vi "bilinear interpolation -- view.vi"() -> ()   [LabVIEW 2010]
uses:
  cursor winow.ctl
  <vilib>/event_ctls.llb/eventvkey.ctl
  cursor window action.ctl
  bylinear interpolation iiii- complex -- build matrix.vi
  Q -- check range -- i -- real.vi
  generate linear region.vi
  line -- complex.vi
  Q -- check range -- i -- integer.vi
  Q - not nan -- real.vi
  Q - not nan -- integer.vi
  Split file name.vi
  <vilib>/Utility/file.llb/Read From Spreadsheet File.vi
  <vilib>/Utility/file.llb/Read From Spreadsheet File (string).vi
  Q regex box.vi
  <vilib>/Analysis/Matrix/Numeric/Conversions/Array To Matrix.vi
  <vilib>/Analysis/Matrix/Numeric/Conversions/Array To Matrix - RA2.vi
  <vilib>/Analysis/baseanly.llb/Inverse Matrix.vi
  <vilib>/Analysis/baseanly.llb/Real Inverse Matrix.vi
  <vilib>/analysis/baseanly.llb/A x B.vi
  <vilib>/Analysis/baseanly.llb/Complex A x B.vi
panel:
  in  "number of segments":i32=3
  out "radius":dbl
  out "circle center":cdb
  in  "scale gauge: Plot: complex plane - filter":dbl(slide)=0.3 min=0.0 max=0.3 step=1e-05 scale=1e-05..0.3 scale format="%#_2g"
  out "Plot: complex plane - filter":cluster{dbl[], dbl[]}[](graph)=[{array[1630 elements], array[1630 elements]}, {[0.4066553079816637, 0.40327728987953354, 0.3931965089365436, 0.37657194509013175, 0.35366577764318885, 0.3248392505398343, 0.2905469753326207, 0.2513297616867779, 0.20780608848872892, 0.16066235006458904, 0.11064203133161113, 0.058533982596904274, 0.005159978916854432, -0.048638239786419776, -0.10201224346646971, -0.15412029220117648, -0.20414061093415437, -0.25128434935829436, -0.29480802255634325, -0.33402523620218605, -0.36831751140939956, -0.39714403851275415, -0.4200502059596971, -0.4366747698061089, -0.44675555074909884, -0.450133568851229, -0.44675555074909884, -0.4366747698061089, -0.420050205959697, -0.3971440385127541, -0.3683175114093995, -0.334025236202186, -0.29480802255634314, -0.25128434935829413, -0.20414061093415412, -0.15412029220117648, -0.10201224346646963, -0.04863823978641969, 0.005159978916854609, 0.05853398259690454, 0.11064203133161105, 0.160662350064589, 0.207806088488729, 0.25132976168677806, 0.2905469753326208, 0.3248392505398345, 0.35366577764318885, 0.3765719450901318, 0.3931965089365437, 0.40327728987953354], [-0.02173913043478265, 0.03195292977291478, 0.08479823411705473, 0.1359633805798755, 0.18464146423708142, 0.23006480263052065, 0.27151704257914155, 0.30834445749658657, 0.33996625704997624, 0.36588374657040623, 0.3856881917657815, 0.399067264704769, 0.40580996941485, 0.40580996941485, 0.39906726470476894, 0.3856881917657815, 0.36588374657040623, 0.33996625704997624, 0.30834445749658657, 0.2715170425791415, 0.23006480263052065, 0.18464146423708136, 0.1359633805798754, 0.08479823411705474, 0.03195292977291471, -0.02173913043478279, -0.07543119064248009, -0.12827649498662014, -0.17944164144944094, -0.22811972510664674, -0.273543063500086, -0.31499530344870685, -0.3518227183661519, -0.38344451791954165, -0.40936200743997164, -0.4291664526353468, -0.4425455255743343, -0.4492882302844153, -0.4492882302844153, -0.44254552557433424, -0.42916645263534686, -0.40936200743997153, -0.38344451791954154, -0.3518227183661518, -0.3149953034487067, -0.27354306350008567, -0.22811972510664671, -0.17944164144944075, -0.12827649498661992, -0.07543119064247988]}, {[-0.08588521013843603, -0.0794706021680707, -0.07305599419770535, -0.06664138622734002, -0.06022677825697468, -0.05381217028660934, -0.04739756231624401, -0.04098295434587867, -0.03456834637551333, -0.02815373840514799, -0.02173913043478265, -0.015324522464417317, -0.008909914494051985, -0.0024953065236866384, 0.003919301446678694, 0.01033390941704404, 0.016748517387409373, 0.023163125357774705, 0.029577733328140052, 0.035992341298505384], [0.4018255934561417, 0.35946912106704926, 0.31711264867795685, 0.2747561762888644, 0.23239970389977196, 0.19004323151067953, 0.14768675912158707, 0.10533028673249467, 0.06297381434340221, 0.020617341954309754, -0.02173913043478265, -0.06409560282387511, -0.10645207521296757, -0.14880854760206003, -0.19116501999115237, -0.23352149238024483, -0.2758779647693373, -0.31823443715842975, -0.3605909095475222, -0.40294738193661456]}, {[0.4018255934561417, 0.35946912106704926, 0.31711264867795685, 0.2747561762888644, 0.23239970389977196, 0.19004323151067953, 0.14768675912158707, 0.10533028673249467, 0.06297381434340221, 0.020617341954309754, -0.02173913043478265, -0.06409560282387511, -0.10645207521296757, -0.14880854760206003, -0.19116501999115237, -0.23352149238024483, -0.2758779647693373, -0.31823443715842975, -0.3605909095475222, -0.40294738193661456], [0.04240694926887073, 0.03599234129850539, 0.029577733328140055, 0.02316312535777472, 0.01674851738740938, 0.01033390941704404, 0.003919301446678708, -0.0024953065236866315, -0.008909914494051971, -0.01532452246441731, -0.02173913043478265, -0.028153738405147982, -0.034568346375513315, -0.04098295434587866, -0.047397562316243994, -0.05381217028660934, -0.06022677825697467, -0.06664138622734, -0.07305599419770535, -0.07947060216807068]}, {[-0.03480491194516355, -0.03153571549706419, -0.02826039650219348, -0.024981001928307045, -0.021699581290264596, -0.018418185369150124, -0.015138864930600241, -0.011863669443142526, -0.008594645797344487, -0.0053338370265733695, -0.002083281030167059, 0.0011549907001868857, 0.004378954350067313, 0.007586595047137542, 0.010775908120375176, 0.01394490035292599, 0.017091591227799845, 0.020214014165629166, 0.023310217753717, 0.02637826696560664], [-0.15235728022815603, -0.15264307469559787, -0.15284705845898403, -0.15296910403510236, -0.15300913514944053, -0.15296712678385516, -0.15284310519220728, -0.1526371478839546, -0.15234938357571062, -0.15197999211080082, -0.15152920434686656, -0.15099730201158656, -0.15038461752660615, -0.14969153379978473, -0.1489184839858907, -0.1480659512158939, -0.1471344682950244, -0.1461246173697867, -0.14503702956413708, -0.14387238458505142]}, {[-0.03913246135316176, -0.03478046636428151, -0.030420320964959106, -0.026054750104140326, -0.021686482121507648, -0.017318247042357023, -0.012952774871420701, -0.008592793886703221, -0.004241028934396603, 9.980027406010505e-05, 0.00442698086171163, 0.008737808481546538, 0.013029589006625965, 0.017299640213825143, 0.021545293460135825, 0.02576389535048096, 0.02995280939600055, 0.03410941766177122, 0.038231122402930216, 0.04231534768818167], [-0.19561963666378376, -0.19600008981485692, -0.19627163553875665, -0.19643410412824466, -0.19648739404574114, -0.19643147198678232, -0.19626637290083468, -0.19599219996945272, -0.19560912454179388, -0.1951173860275308, -0.19451729174722807, -0.19380921674027698, -0.19299360353050807, -0.1920709618496281, -0.1910418683186543, -0.1899069660875451, -0.18866696443325223, -0.1873226383164459, -0.18587482789718943, -0.1843244380098665]}]
  in  "cursor bracket: All, data window":T1={"left"=2889.388009121066, "right "=2961.3698154668923, "center"=2923.047912677266, "window"=71.98180634582651, "cursors"=[0, 1, 2], "relative"=1, "absolute"=1, "fixed vertical offset"=2421.6740576496672, "vertical offset"=2421.6740576496672, "skew"=0.0, "default window frac"=0.0, "kind"=enum."symmetric", "skew.left"=0.3, "skew.right"=1.0, "Plot ref"=refnum, "wing order"=enum."back"}
  out "Plot: All":cluster{"all rows":dbl[], "all rows":dbl[]}[](graph)
  in  "phase is normalized":bool=TRUE
  in  "filter  all":bool
  out "all:min omega":dbl=450.0
  out "all:max omega":dbl=3099.911666666456
  in  "read freq in":bool=TRUE
  in  "# columns in bin file":i32=3
  in  "create bin file from dat":bool=TRUE
  out "Char":i16
  in  "file path":path=path "C:/data/RUS/Experiment/ProbeTest/Probe10/Hg1201-4-C199-80K-1/Sweep1/March_2012/032212/201.57400K_900_2100_001_032212.bin"
  out "Numeric":i32
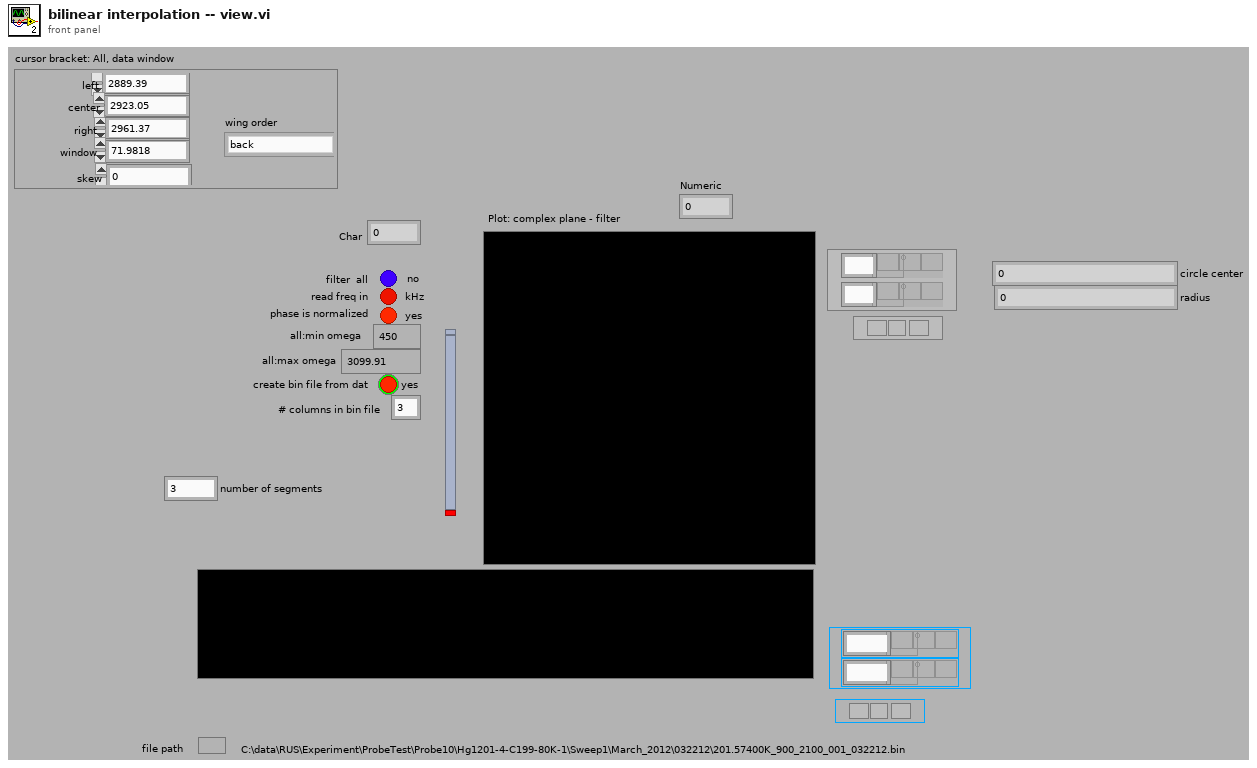
[diagram p1: front panel]
types:
  T1 = typedef "cursor winow.ctl" = cluster{"left":dbl, "right ":dbl, "center":dbl, "window":dbl, "cursors":i32[], "relative":i32, "absolute":i32, "fixed vertical offset":dbl, "vertical offset":dbl, "skew":dbl, "default window frac":dbl, "kind":enum16{"symmetric", "skewed", "fancy"}, "skew.left":dbl, "skew.right":dbl, "Plot ref":refnum<vi>, "wing order":enum16{"forw", "back"}}
  T2 = typedef "eventvkey.ctl" = enum16{"ASCII", "Enter", "Return", "Shift", "Ctrl", "Alt", "Cmd", "Opt", "Caps", "NumLock", "Clear", "Break", "Up", "Down", "Left", "Right", "Insert", "Delete", "Home", "End", "PageUp", "PageDown", "Escape", "Help", "Pause", "ScrollLock", "F1", "F2", "F3", "F4", "F5", "F6", "F7", "F8", "F9", "F10", "F11", "F12", "F13", "F14", "F15", "F16", "F17", "F18", "F19", "F20", "F21", "F22", "F23", "F24", "Play", "VolumeUp", "VolumeDown", "Mute", "Two Byte Char"}
  T3 = typedef "cursor window action.ctl" = enum16{"balance", "h. offset change", "cursor moves", "change center", "change window", "init", "check", "reset", "set y to middle", "idle", "-write all Y", "-write left.X", "-write center.X", "-write right.X", "-write all X", "-change center", "-change window", "-change skew", "-read cursor 2", "-read cursor 1", "-read cursor 0", "-read all cursors", "-reset", "-read plot scale", "-set y to middle", "-Q: center.Y is visible", "-Q: window is visible", "-parse center.Y", "-right left from center", "-left move", "-right move", "-set center.Y", "-empty", "-set cursors to default", "-check", "-write center.Y", "-copy cursor 1", "-copy cursor 0", "-copy cursor 2", "move right", "move left", "shrink", "broaden", "skew up", "skew down", "-write plot scale", "zoom X", "change cen&win"}
  T4 = cluster{"left":dbl, "right ":dbl, "center":dbl, "window":dbl, "cursors":i32[], "relative":i32, "absolute":i32, "fixed vertical offset":dbl, "vertical offset":dbl, "skew":dbl, "default window frac":dbl, "kind":enum16{"symmetric", "skewed", "fancy"}, "skew.left":dbl, "skew.right":dbl, "Plot ref":refnum<vi>, "wing order":enum16{"forw", "back"}}
  T5 = typedef "lveventtype.ctl" = enum32{"Null", "Timeout", "App Instance Close", "App Instance Close?", "Autoscale Range Change", "Cell Edit", "Cell Edit?", "Cursor Grab", "Cursor Grab?", "Cursor Move", "Cursor Release", "Data Change", "Direction Change", "Display State Change", "Drag Ended", "Drag Enter", "Drag Leave", "Drag Over", "Drag Source Update", "Drag Starting", "Drag Starting?", "Drop", "Exec State Change", "Key Down", "Key Down?", "Key Repeat", "Key Repeat?", "Key Up", "Listbox Double Click", "Menu Activation?", "Menu Selection (App)", "Menu Selection? (App)", "Menu Selection (User)", "Mouse Down", "Mouse Down?", "Mouse Enter", "Mouse Leave", "Mouse Move", "Mouse Up", "NI Security User Change (App)", "Pane Size", "Panel Close", "Panel Close?", "Panel Resize", "Plot Attribute Change", "Scale Range Change", "Shortcut Menu Activation?", "Shortcut Menu Selection (App)", "Shortcut Menu Selection? (App)", "Shortcut Menu Selection (User)", "Tree Double Click", "Tree Drag", "Tree Drag?", "Tree Drop", "Tree Drop?", "Tree Item Close", "Tree Item Close?", "Tree Item Open", "Tree Item Open?", "Value Change"}
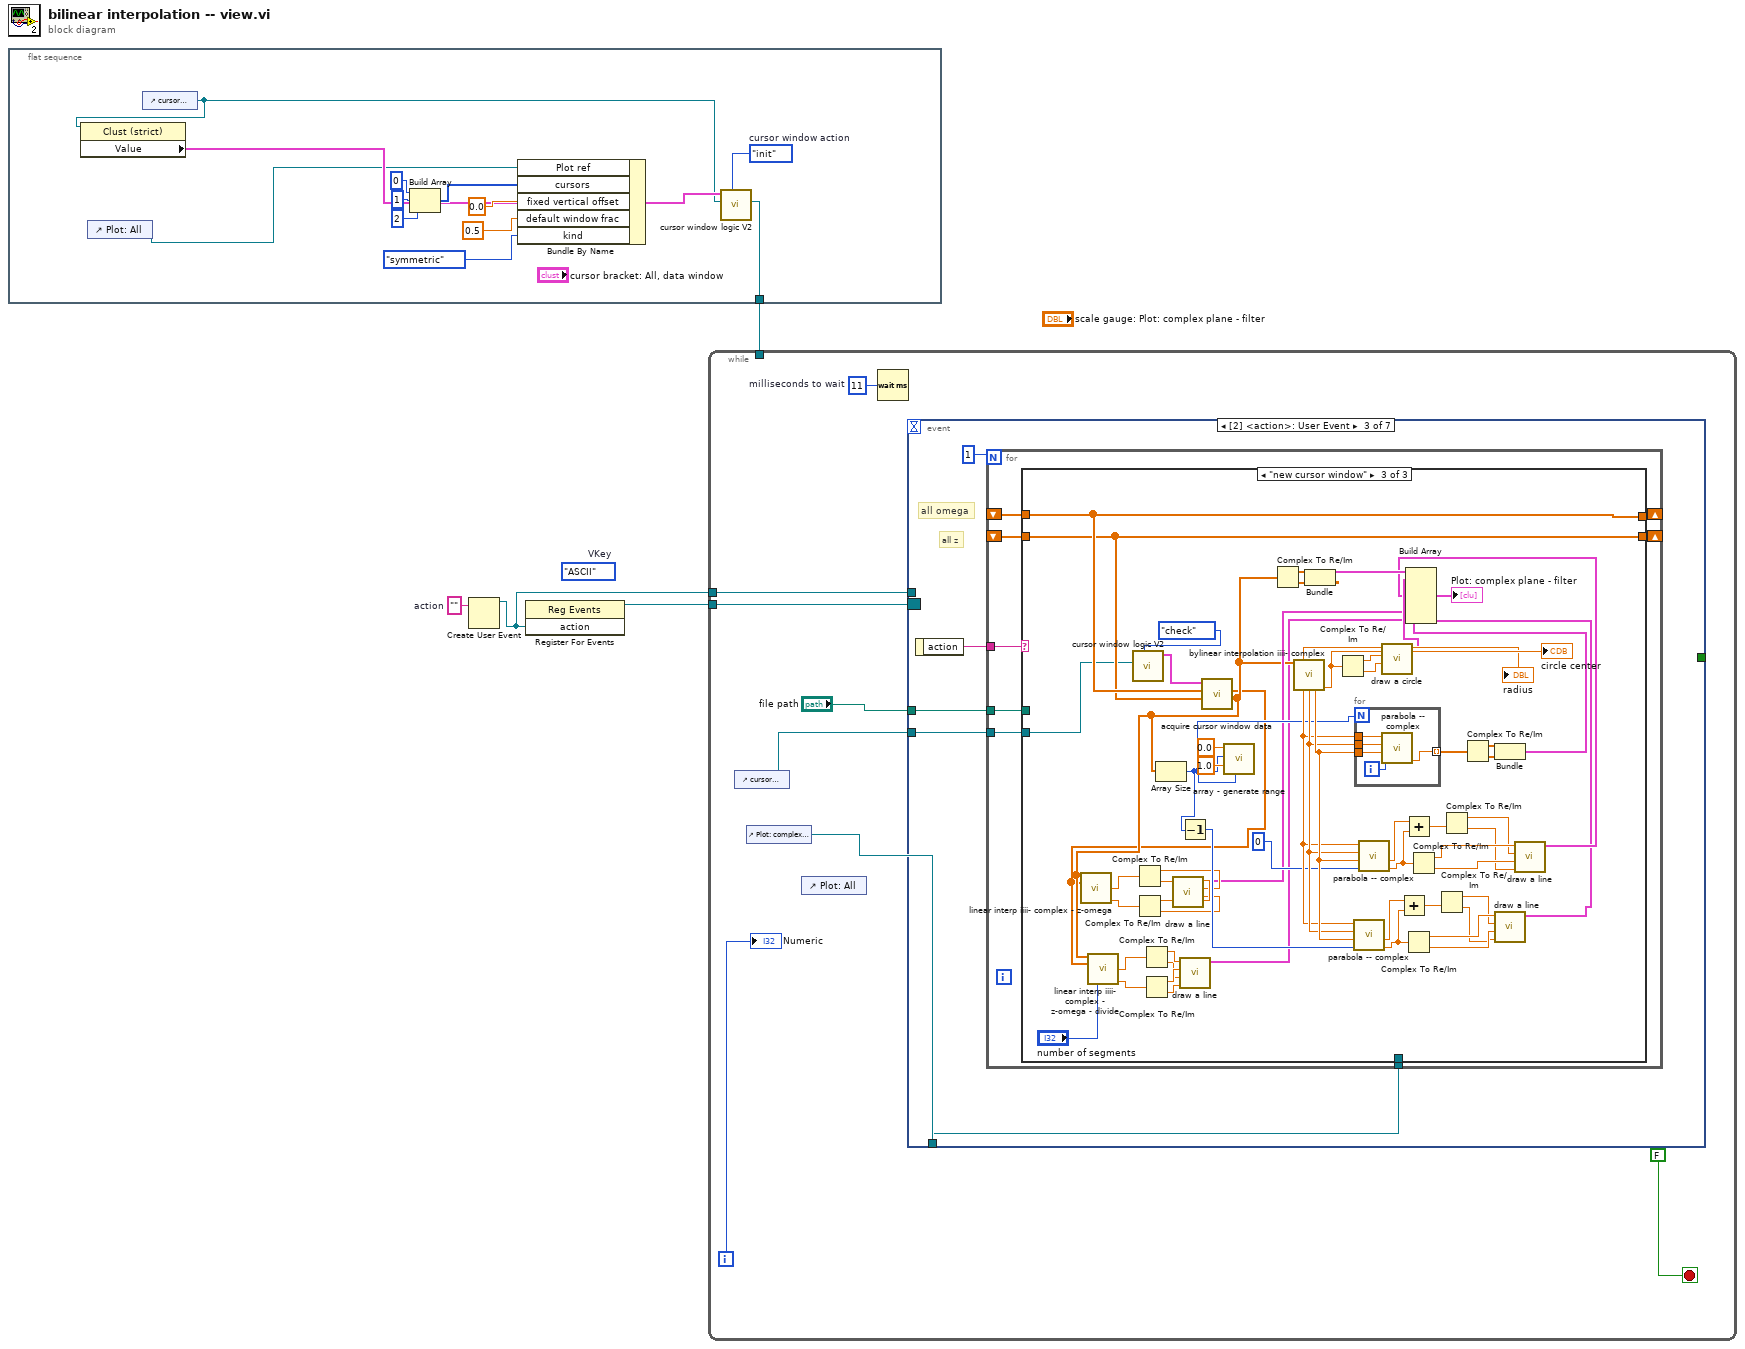
[diagram p0: block diagram]
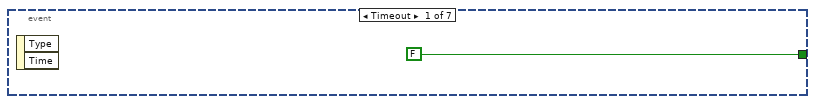
[diagram p2: hidden frame]
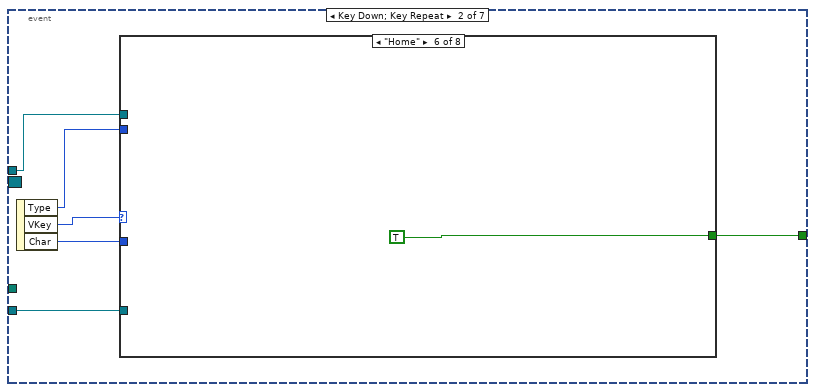
[diagram p3: hidden frame]
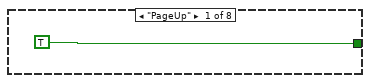
[diagram p4: hidden frame]
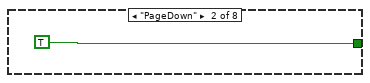
[diagram p5: hidden frame]
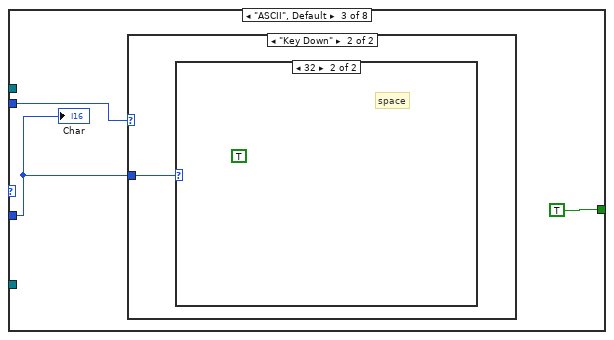
[diagram p6: hidden frame]
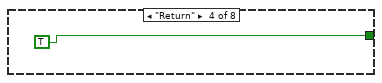
[diagram p9: hidden frame]
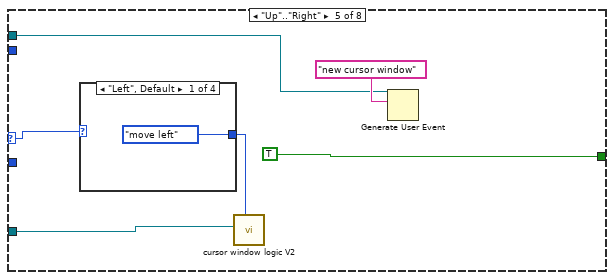
[diagram p10: hidden frame]
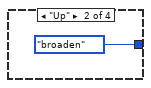
[diagram p11: hidden frame]
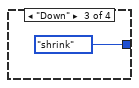
[diagram p12: hidden frame]
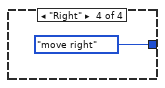
[diagram p13: hidden frame]
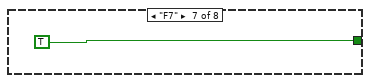
[diagram p14: hidden frame]
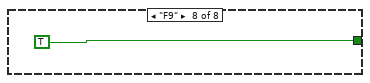
[diagram p15: hidden frame]
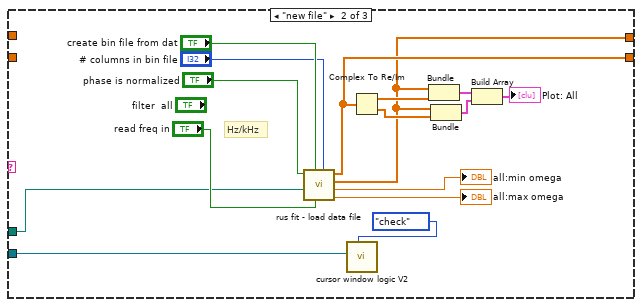
[diagram p17: hidden frame]
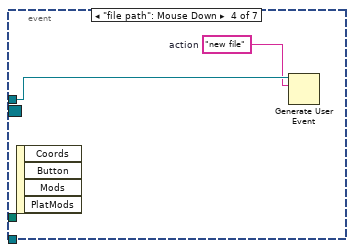
[diagram p18: hidden frame]
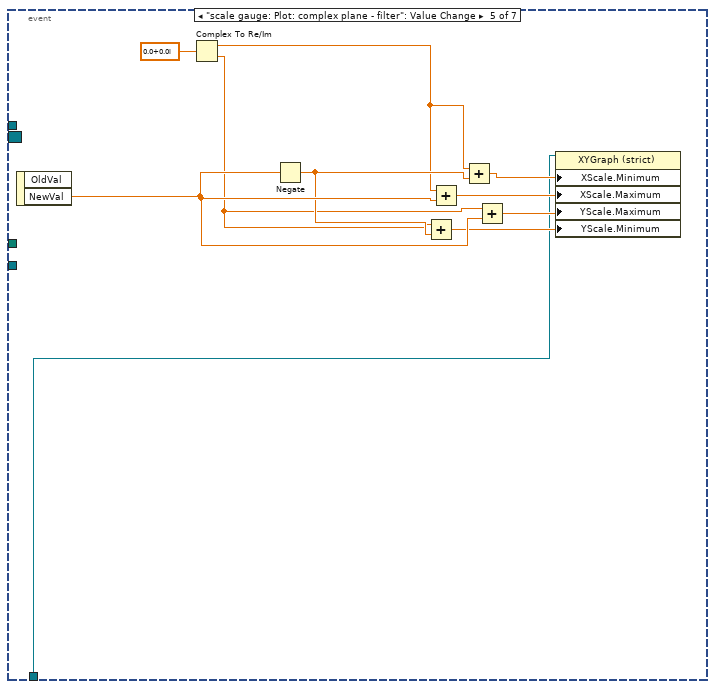
[diagram p19: hidden frame]
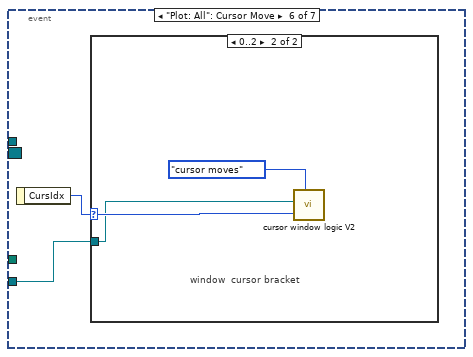
[diagram p20: hidden frame]
diagram:
  (unwired) eventvkey."ASCII"  # VKey
  w3 = ""  # action
  n1 = flat-sequence {
    tunnel: [w5] -> w2
    frame #0 {
      w8 = cursor_window_action."init"  # cursor window action
      n2 = control-ref of="Plot: All"() -> (w7:refnum<vi>)
      n3 = control-ref of="cursor bracket: All, data window"() -> (w6:refnum<vi>)
      n4 = property class="Clust (strict)"(reference=w6) -> ("Value"=w9:T4)  [unwired: 1 in, 2 out]
      n5 = Build Array(0, 1, 2) -> (w16:i32[])
      n6 = Bundle By Name(cluster=w9, "Plot ref"=w7, "cursors"=w16, "fixed vertical offset"=0.0, "default window frac"=0.5 ("fixed vertical offset"), "kind"=enum16{"symmetric", "skewed", "fancy"}."symmetric") -> (w17:T4)
      n7 = call "cursor window logic V2.vi"("cursor window action"=w8, "cursor window in"=w6, "cursor window init"=w17) -> ("cursor window out"=w5:refnum<vi>)  [unwired: 7 in, 1 out]
    }
  }
  n8 = Create User Event(user event datatype=w3) -> (user event=w1:refnum<user-event>)  [unwired: 1 in, 1 out]
  n9 = register-events(w1) -> (reference out=w4:refnum<event-registration>)  [unwired: 2 in, 1 out]
  n10 = while {
    tunnel: w4 -> [w25]
    tunnel: w2 -> [_]
    tunnel: w1 -> [w20]
    i -> [w18]
    stop <- FALSE stop-if-true
    w24 = u32 11  # milliseconds to wait
    n11 = control-ref of="cursor bracket: All, data window"() -> (w21:refnum<vi>)
    n12 = control-ref of="Plot: complex plane - filter"() -> (w19:refnum<vi>)
    n13 = control-ref of="Plot: All"() -> ()  [unwired: 1 out]
    n14 = Wait (ms)(milliseconds to wait=w24) -> ()  [unwired: 1 out]
    n15 = event shown="[2] <action>: User Event" {
      selector: w25 -> [_ _ _ _ _ _ _]
      dyn-events: _ -> [_ _ _ _ _ _ _]
      timeout: _ -> [_ _ _ _ _ _ _]
      tunnel: [FALSE w30 _ _ _ _ _] -> _
      tunnel: "file path" -> [_ _ w56 _ _ _ _]
      tunnel: w21 -> [_ w28 w55 _ _ w160 _]
      tunnel: w20 -> [_ w27 _ w149 _ _ w165]
      tunnel: w19 -> [_ _ w53 _ w151 _ _]
      event Timeout {
        n16 = event-data() -> ()  [unwired: 1 in, 2 out]
      }
      event Key Down; Key Repeat {
        n17 = event-data() -> ("Type"=w29:T5, "VKey"=w32:T2, "Char"=w31:i16)  [unwired: 1 in]
        n18 = case shown="\"Home\"" w32 {
          selector: w32 -> [_ _ _ _ w40 _ _ _]
          tunnel: w31 -> [_ _ w36 _ _ _ _ _]
          tunnel: [TRUE TRUE TRUE TRUE TRUE TRUE TRUE TRUE] -> w30
          tunnel: w29 -> [_ _ w35 _ _ _ _ _]
          tunnel: w28 -> [_ _ _ _ w44 _ _ _]
          tunnel: w27 -> [_ _ _ _ w41 _ _ _]
          frame "PageUp" {
          }
          frame "PageDown" {
          }
          frame "ASCII", Default {
            n19 = case shown="\"Key Down\"" w35 {
              tunnel: w36 -> [_ w38]
              frame "Null", Default {
              }
              frame "Key Down" {
                n20 = case shown="32" w38 {
                  frame 0, Default {
                  }
                  frame 32 {
                    (unwired) TRUE
                    # "space"
                  }
                }
              }
            }
            "Char" <- w36
          }
          frame "Return" {
          }
          frame "Up".."Right" {
            n21 = case shown="\"Left\", Default" w40 {
              tunnel: [cursor_window_action."move left" ("cursor window action") cursor_window_action."broaden" ("cursor window action") cursor_window_action."shrink" ("cursor window action") cursor_window_action."move right" ("cursor window action")] -> w43
              frame "Left", Default {
              }
              frame "Up" {
              }
              frame "Down" {
              }
              frame "Right" {
              }
            }
            n22 = call "cursor window logic V2.vi"("cursor window action"=w43, "cursor window in"=w44) -> ()  [unwired: 8 in, 2 out]
            n23 = Generate User Event(user event=w41, event data cluster="new cursor window" ("event data")) -> ()  [unwired: 1 in, 2 out]
          }
          frame "Home" {
          }
          frame "F7" {
          }
          frame "F9" {
          }
        }
      }
      event User Event {
        # "all z"
        # "all omega"
        n24 = event-data() -> ("action"=w57:string)  [unwired: 1 in]
        n25 = for {
          N: 1 -> [_]
          tunnel: w57 -> [w65]
          tunnel: w56 -> [w64]
          shift-right: [w63] -> _
          shift-left: _ -> [w60]
          shift-right: [w62] -> _
          shift-left: _ -> [w61]
          tunnel: w55 -> [w59]
          tunnel: w53 -> [w58]
          n26 = case shown="\"new cursor window\"" w65 {
            tunnel: w64 -> [_ w72 _]
            tunnel: [w66 w71 w139] -> w63
            tunnel: [w67 w70 w140] -> w62
            tunnel: w61 -> [w67 _ w140]
            tunnel: w60 -> [w66 _ w139]
            tunnel: w59 -> [_ w68 w138]
            tunnel: w58 -> [_ _ _]
            frame "False", Default {
            }
            frame "new file" {
              # "Hz/kHz"
              n27 = call "rus fit - load data file.vi"("number of columns in the binary file"="# columns in bin file", "read freq in"="read freq in", "create bin file when only dat file is present"="create bin file from dat", "file path"=w72, "phase is normalized"="phase is normalized") -> ("all:max omega"=→"all:max omega":dbl, "all:min omega"=→"all:min omega":dbl, "omega"=w70:dbl[], "x + iy"=w71:cdb[])  [unwired: 2 in, 1 out]
              n28 = call "cursor window logic V2.vi"("cursor window action"=cursor_window_action."check", "cursor window in"=w68) -> ()  [unwired: 8 in, 2 out]
              n29 = Complex To Re/Im(x + iy=w71) -> (x=w80:dbl[], y=w79:dbl[])
              n30 = Bundle("omega"=w70, w80) -> (w81:cluster{"omega":dbl[], dbl[]})  [unwired: 1 in]
              n31 = Bundle("omega"=w70, w79) -> (w82:cluster{"omega":dbl[], dbl[]})  [unwired: 1 in]
              n32 = Build Array(w81, w82) -> (→"Plot: All":cluster{"omega":dbl[], dbl[]}[])
            }
            frame "new cursor window" {
              n33 = call "cursor window logic V2.vi"("cursor window action"=cursor_window_action."check", "cursor window in"=w138) -> ("cursor window out"=w141:T1)  [unwired: 8 in, 1 out]
              n34 = call "acquire cursor window data.vi"("z in"=w139, "omega in"=w140, "cursor window"=w141) -> ("z out"=w91:cdb[], "omega  out"=w85:dbl[])  [unwired: 7 in]
              n35 = call "linear interp iiii- complex - z-omega.vi"("z"=w91, "omega"=w85) -> ("left"=w96:cdb, "right"=w95:cdb)  [unwired: 5 in, 7 out]
              n36 = call "linear interp iiii- complex - z-omega - divide.vi"("z"=w91, "number of segments"="number of segments", "omega"=w85) -> ("left"=w93:cdb, "right"=w92:cdb)  [unwired: 3 in, 8 out]
              n37 = Complex To Re/Im(x + iy=w96) -> (x=w99:dbl, y=w97:dbl)
              n38 = Complex To Re/Im(x + iy=w95) -> (x=w100:dbl, y=w98:dbl)
              n39 = Complex To Re/Im(x + iy=w93) -> (x=w90:dbl, y=w88:dbl)
              n40 = Complex To Re/Im(x + iy=w92) -> (x=w89:dbl, y=w87:dbl)
              n41 = Array Size(array=w91) -> (size(s)=w103:i32)
              n42 = call "draw a line.vi"("y1"=w97, "y0"=w98, "x1"=w99, "x0"=w100) -> ("output cluster"=w94:cluster{dbl[], dbl[]})  [unwired: 7 in]
              n43 = Decrement(x=w103) -> (x-1=w102:i32)
              n44 = call "draw a line.vi"("y1"=w87, "y0"=w88, "x1"=w89, "x0"=w90) -> ("output cluster"=w86:cluster{dbl[], dbl[]})  [unwired: 7 in]
              n45 = call "array - generate range.vi"("N"=w103, "df"=1.0, "freq max"=w103, "freq min"=0.0) -> ()  [unwired: 7 in, 1 out]
              n46 = Complex To Re/Im(x + iy=w91) -> (x=w137:dbl[], y=w136:dbl[])
              n47 = call "bylinear interpolation iiii- complex.vi"("Array"=w91) -> ("radius"=w130:dbl, "intercept"=w109:cdb, "slope"=w110:cdb, "curvature"=w111:cdb, "circle center"=w133:cdb)  [unwired: 4 in, 6 out]
              "circle center" <- w133
              "radius" <- w130
              n48 = Bundle(w137, w136) -> (w135:cluster{dbl[], dbl[]})  [unwired: 1 in]
              n49 = Complex To Re/Im(x + iy=w133) -> (x=w132:dbl, y=w131:dbl)
              n50 = call "parabola -- complex.vi"("n"=w102, "curvature"=w111, "slope"=w110, "intercept"=w109) -> ("parabola"=w114:cdb, "tangent"=w113:cdb)  [unwired: 6 in]
              n51 = for {
                N: w103 -> [_]
                tunnel: w109 -> [w147]
                tunnel: w110 -> [w146]
                tunnel: w111 -> [w145]
                tunnel: [w143] -> w125 mode=indexing
                i -> [w144]
                n52 = call "parabola -- complex.vi"("n"=w144, "curvature"=w145, "slope"=w146, "intercept"=w147) -> ("parabola"=w143:cdb)  [unwired: 6 in, 1 out]
              }
              n53 = call "parabola -- complex.vi"("n"=0, "curvature"=w111, "slope"=w110, "intercept"=w109) -> ("parabola"=w122:cdb, "tangent"=w121:cdb)  [unwired: 6 in]
              n54 = call "draw a circle.vi"("center Y"=w131, "center x"=w132, "radius"=w130) -> ("output cluster"=w129:cluster{dbl[], dbl[]})  [unwired: 8 in]
              n55 = Add(x=w113, y=w114) -> (x+y=w112:cdb)
              n56 = Add(x=w121, y=w122) -> (x+y=w120:cdb)
              n57 = Complex To Re/Im(x + iy=w114) -> (x=w108:dbl, y=w106:dbl)
              n58 = Complex To Re/Im(x + iy=w122) -> (x=w119:dbl, y=w117:dbl)
              n59 = Complex To Re/Im(x + iy=w112) -> (x=w107:dbl, y=w105:dbl)
              n60 = Complex To Re/Im(x + iy=w120) -> (x=w118:dbl, y=w116:dbl)
              n61 = Complex To Re/Im(x + iy=w125) -> (x=w126:dbl[], y=w124:dbl[])
              n62 = Bundle(w126, w124) -> (w123:cluster{dbl[], dbl[]})  [unwired: 1 in]
              n63 = call "draw a line.vi"("y1"=w105, "y0"=w106, "x1"=w107, "x0"=w108) -> ("output cluster"=w104:cluster{dbl[], dbl[]})  [unwired: 7 in]
              n64 = call "draw a line.vi"("y1"=w116, "y0"=w117, "x1"=w118, "x0"=w119) -> ("output cluster"=w115:cluster{dbl[], dbl[]})  [unwired: 7 in]
              n65 = Build Array(w135, w129, w123, w115, w104, w94, w86) -> (→"Plot: complex plane - filter":cluster{dbl[], dbl[]}[])
            }
          }
        }
      }
      event "file path": Mouse Down {
        w148 = "new file"  # action
        n66 = event-data() -> ()  [unwired: 1 in, 4 out]
        n67 = Generate User Event(user event=w149, event data cluster=w148) -> ()  [unwired: 1 in, 2 out]
      }
      event "scale gauge: Plot: complex plane - filter": Value Change {
        n68 = event-data() -> ("NewVal"=w159:dbl)  [unwired: 1 in, 1 out]
        n69 = Complex To Re/Im(x + iy=cdb 0.0+0.0i) -> (x=w152:dbl, y=w153:dbl)
        n70 = Negate(x=w159) -> (-x=w158:dbl)
        n71 = Add(x=w153, y=w158) -> (x+y=w154:dbl)
        n72 = Add(x=w152, y=w159) -> (x+y=w156:dbl)
        n73 = Add(x=w152, y=w158) -> (x+y=w157:dbl)
        n74 = Add(x=w153, y=w159) -> (x+y=w155:dbl)
        n75 = property on="Property Node" class="XYGraph (strict)"(reference=w151, "XScale.Minimum"=w157, "XScale.Maximum"=w156, "YScale.Maximum"=w155, "YScale.Minimum"=w154) -> ()  [unwired: 1 in, 2 out]
      }
      event "Plot: All": Cursor Move {
        n76 = event-data() -> ("CursIdx"=w161:i32)  [unwired: 1 in]
        n77 = case shown="0..2" w161 {
          selector: w161 -> [_ w164]
          tunnel: w160 -> [_ w162]
          frame 3..5, Default {
          }
          frame 0..2 {
            # "window  cursor bracket"
            n78 = call "cursor window logic V2.vi"("CursIdx"=w164, "cursor window action"=cursor_window_action."cursor moves", "cursor window in"=w162) -> ()  [unwired: 7 in, 2 out]
          }
        }
      }
      event "Plot: All": Cursor Release {
        n79 = event-data() -> ()  [unwired: 1 in, 1 out]
        n80 = Generate User Event(user event=w165, event data cluster="new cursor window" ("event data")) -> ()  [unwired: 1 in, 2 out]
      }
    }
    "Numeric" <- w18
  }
